vi "ReadMultiple.vi"(8 "error in (no error)":errorcluster, 11 "Agilent DSO-X 3032A in":refnum<class "Agilent DSO-X 3032A.lvclass">) -> (0 "error out":errorcluster, 1 "timed out?":bool, 2 "Data":refnum<class "AbstractData.lvclass">, 3 "Agilent DSO-X 3032A out":refnum<class "Agilent DSO-X 3032A.lvclass">)   [LabVIEW 2014, in "Agilent DSO-X 3032A.lvclass"]
uses:
  Agilent DSO-X 3032A.lvclass
  Framework/Model/Data/Data1D/Data1D.lvclass
  Framework/Interfaces/Observable Actor/Observable Actor.lvclass
  Framework/Model/Data/AbstractData/AbstractData.lvclass
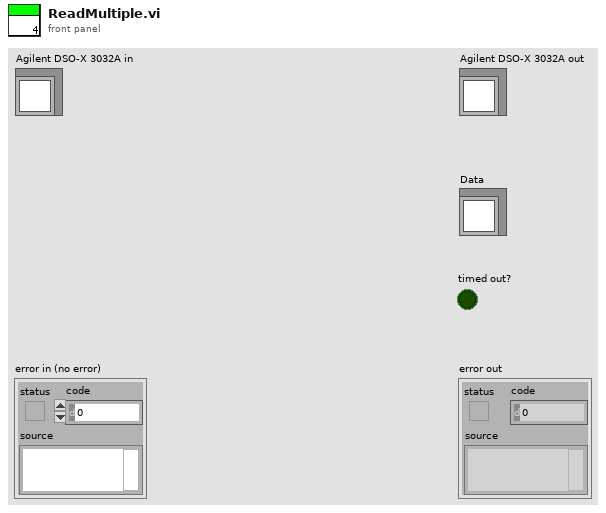
[diagram p1: front panel]
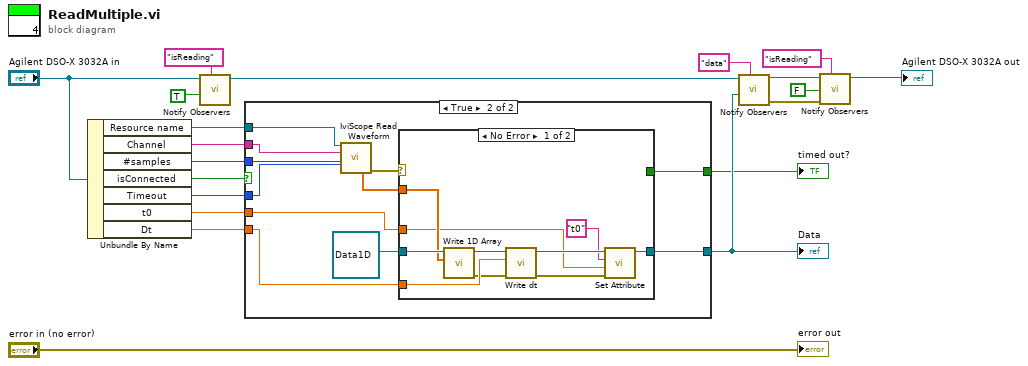
[diagram p0: block diagram]
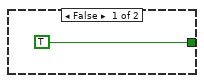
[diagram p2: hidden frame]
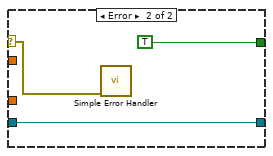
[diagram p3: hidden frame]
diagram:
  n1 = Unbundle By Name("Agilent DSO-X 3032A in") -> ("Resource name"=w19:refnum<k15>, "Channel"=w14:string, "#samples"=w20:i32, "isConnected"=w18:bool, "Timeout"=w17:i32, "t0"=w12:dbl, "Dt"=w11:dbl)
  n2 = call "Notify Observers.vi"("name"="isReading", "value"=TRUE, "Observable Actor in"="Agilent DSO-X 3032A in") -> ("Observable Actor out"=w1:refnum<class "Agilent DSO-X 3032A.lvclass">)  [unwired: 7 in, 1 out]
  n3 = case shown="True" w18 {
    tunnel: [_ w26] -> w16
    tunnel: w20 -> [_ w30]
    tunnel: w19 -> [_ w32]
    tunnel: w17 -> [_ w22]
    tunnel: w14 -> [_ w31]
    tunnel: [TRUE w25] -> w13
    tunnel: w12 -> [_ w23]
    tunnel: w11 -> [_ w24]
    frame False {
    }
    frame True {
      n4 = call <vilib>:"IviScope Read Waveform.vi"("instrument handle"=w32, "channel name (\"CHANNEL1\")"=w31, "waveform size (0)"=w30, "maximum time (5000ms)"=w22) -> ("waveform array"=w28:dbl[], "error out"=w29:errorcluster)  [unwired: 6 in, 4 out]
      n5 = case shown="No Error" w29 {
        selector: w29 -> [_ w43]
        tunnel: w28 -> [w40 _]
        tunnel: refnum<class "Data1D.lvclass"> refnum ("Data1D.lvclass") -> [w42 w45]
        tunnel: [w36 w45] -> w26
        tunnel: w24 -> [w39 _]
        tunnel: [_ TRUE] -> w25
        tunnel: w23 -> [w33 _]
        frame No Error {
          n6 = call "Write 1D Array.vi"("1D Array"=w40, "Data1D in"=w42) -> ("error out"=w38:errorcluster, "Data1D out"=w41:refnum<class "Data1D.lvclass">)  [unwired: 8 in]
          n7 = call "Write dt.vi"("error in (no error)"=w38, "dt"=w39, "Data1D in"=w41) -> ("error out"=w34:errorcluster, "Data1D out"=w37:refnum<class "Data1D.lvclass">)  [unwired: 7 in]
          n8 = call-dynamic "Set Attribute.vi"("error in (no error)"=w34, "Value"=w33, "Name"="t0", "AbstractData in"=w37) -> ("AbstractData out"=w36:refnum<class "Data1D.lvclass">)  [unwired: 5 in, 2 out]
        }
        frame Error {
          n9 = call <vilib>:"Simple Error Handler.vi"("error in (no error)"=w43) -> ()  [unwired: 4 in, 5 out]
        }
      }
    }
  }
  "Data" <- w16
  "timed out?" <- w13
  n10 = call "Notify Observers.vi"("name"="data", "value"=w16, "Observable Actor in"=w1) -> ("error out"=w7:errorcluster, "Observable Actor out"=w8:refnum<class "Agilent DSO-X 3032A.lvclass">)  [unwired: 7 in]
  n11 = call "Notify Observers.vi"("name"="isReading", "error in (no error)"=w7, "value"=FALSE, "Observable Actor in"=w8) -> ("Observable Actor out"=→"Agilent DSO-X 3032A out":refnum<class "Agilent DSO-X 3032A.lvclass">)  [unwired: 6 in, 1 out]
  "error out" <- "error in (no error)"
